vi "GA Home Get Prm Single.vi"(0 "iAxisNum":i16, 1 "nHomeMode":i16, 2 "nHomeDir":i16, 3 "lOffset":i32, 4 "dHomeRapidVel":dbl, 5 "dHomeLocatVel":dbl, 6 "dHomeIndexVel":dbl, 7 "error in (no error)":errorcluster caption="错误输入（无错误）", 8 "dHomeAcc":dbl) -> (18 "dHomeAcc out":dbl, 20 "function return":i32, 21 "nHomeMode out":i16, 22 "nHomeDir out":i16, 23 "lOffset out":i32, 24 "dHomeRapidVel out":dbl, 25 "dHomeLocatVel out":dbl, 26 "dHomeIndexVel out":dbl, 27 "error out":errorcluster caption="错误输出")   [LabVIEW 2015, in "GAS.lvlib"]
doc: "extern \"C\" __declspec(dllimport) int GA_HomeGetPrmSingle(short iAxisNum,short *nHomeMode,short *nHomeDir,long *lOffset,double* dHomeRapidVel,double* dHomeLocatVel,double* dHomeIndexVel,double* dHomeAcc);"
uses:
  <userlib>/BP_GAS/GAS.lvlib
  <userlib>/BP_GAS/GAS.dll
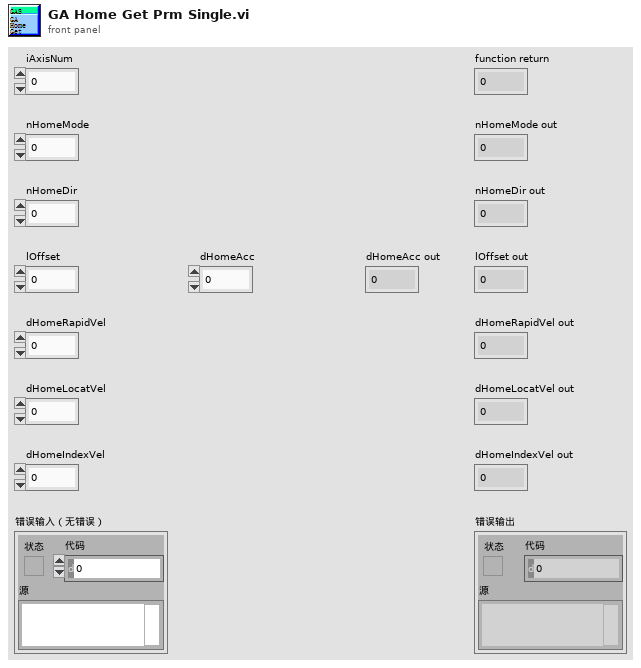
[diagram p1: front panel]
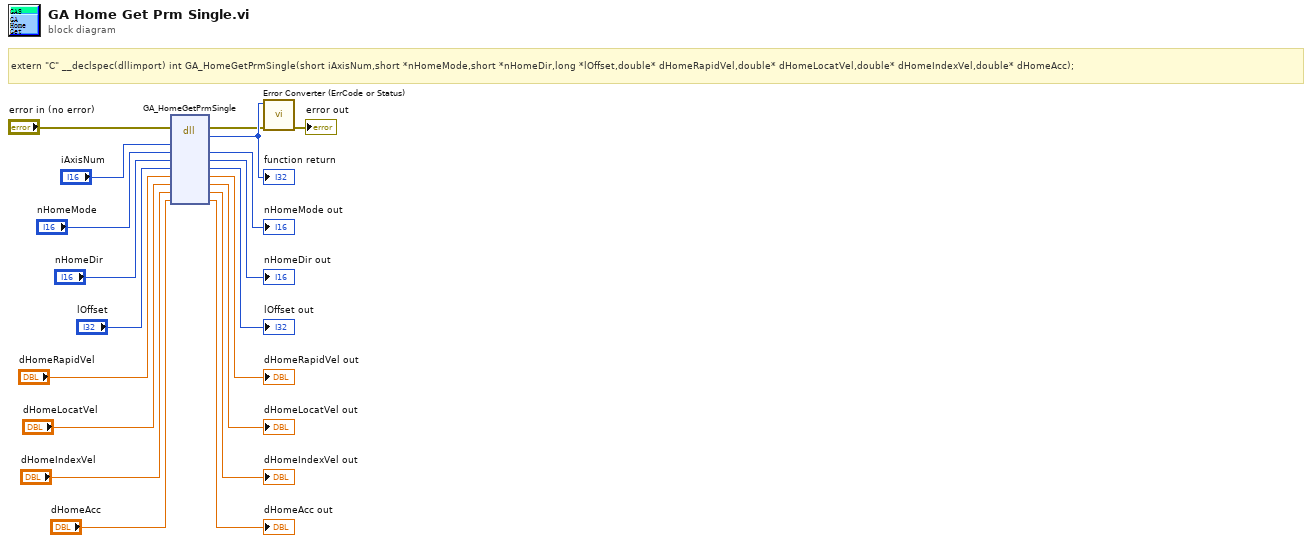
[diagram p0: block diagram]
diagram:
  # "extern \"C\" __declspec(dllimport) int GA_HomeGetPrmSingle(short iAxisNum,short *nHomeMode,short *nHomeDir,long *lOffset,double* dHomeRapidVel,double* dHomeLocatVel,double* dHomeIndexVel,double* dHomeAcc);"
  n1 = dll-call lib="E:/Program Files (x86)/National Instruments/LabVIEW 2015/user.lib/BP_GAS/GAS.*" fn="GA_HomeGetPrmSingle"(error in="error in (no error)", "iAxisNum"="iAxisNum", "nHomeMode"="nHomeMode", "nHomeDir"="nHomeDir", "lOffset"="lOffset", "dHomeRapidVel"="dHomeRapidVel", "dHomeLocatVel"="dHomeLocatVel", "dHomeIndexVel"="dHomeIndexVel", "dHomeAcc"="dHomeAcc") -> (error out=w2:errorcluster, w19:i32, "nHomeMode"=→"nHomeMode out":i16, "nHomeDir"=→"nHomeDir out":i16, "lOffset"=→"lOffset out":i32, "dHomeRapidVel"=→"dHomeRapidVel out":dbl, "dHomeLocatVel"=→"dHomeLocatVel out":dbl, "dHomeIndexVel"=→"dHomeIndexVel out":dbl, "dHomeAcc"=→"dHomeAcc out":dbl)  [unwired: 3 in, 1 out]
  "function return" <- w19
  n2 = call "Error Converter (ErrCode or Status).vi"("error in (no error)"=w2, "error code"=w19) -> ("error out"=→"error out":errorcluster)  [unwired: 9 in]
